vi "执行文件路径修正.vi"(4 "Path":path) -> (2 "Path out":path)   [LabVIEW 2013]
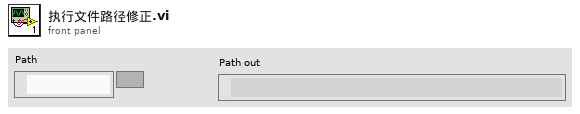
[diagram p1: front panel]
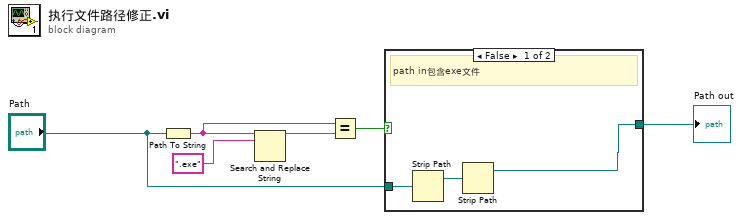
[diagram p0: block diagram]
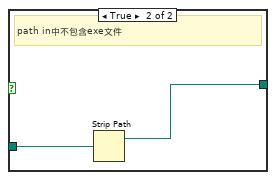
[diagram p2: hidden frame]
diagram:
  n1 = Path To String(path="Path") -> (string=w4:string)
  n2 = Search and Replace String(input string=w4, search string=".exe") -> (result string=w5:string)  [unwired: 6 in, 3 out]
  n3 = Equal?(x=w4, y=w5) -> (x = y?=w2:bool)
  n4 = case shown="False" w2 {
    tunnel: [w7 w10] -> w3
    tunnel: "Path" -> [w9 w11]
    frame False {
      # "path in包含exe文件"
      n5 = Strip Path(path=w9) -> (stripped path=w8:path)  [unwired: 1 out]
      n6 = Strip Path(path=w8) -> (stripped path=w7:path)  [unwired: 1 out]
    }
    frame True {
      # "path in中不包含exe文件"
      n7 = Strip Path(path=w11) -> (stripped path=w10:path)  [unwired: 1 out]
    }
  }
  "Path out" <- w3
